vi "FreqC.Close Session.vi"(8 "error In":errorcluster, 11 "FreqC Session in":T1) -> (0 "error out":errorcluster)   [LabVIEW 2018]
uses:
  typedefs/FreqC.Session.ctl
  <instrlib>/Agilent 532XX Series/Agilent 532XX Series.lvlib
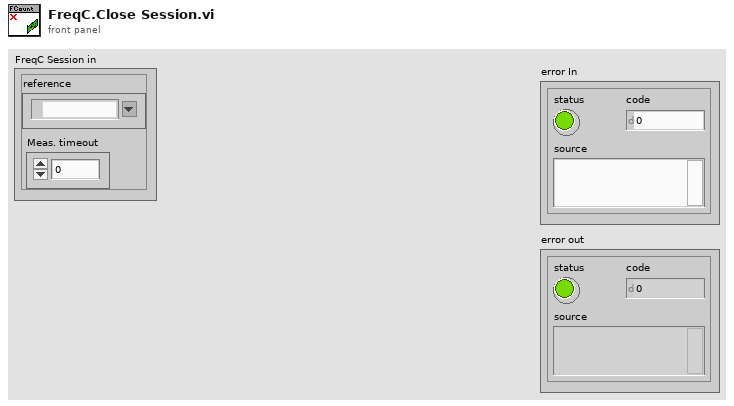
[diagram p1: front panel]
types:
  T1 = typedef "FreqC.Session.ctl" = cluster{"reference":refnum<visa-resource-name>, "Meas. timeout":dbl}
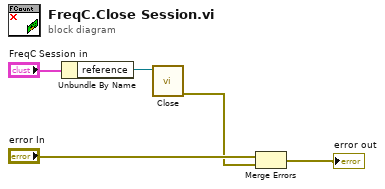
[diagram p0: block diagram]
diagram:
  n1 = Unbundle By Name("FreqC Session in") -> ("reference"=w4:refnum<visa-resource-name>)
  n2 = call <instrlib>:"Close.vi"("VISA resource name"=w4) -> ("error out"=w2:errorcluster)  [unwired: 10 in]
  n3 = Merge Errors("error In", w2) -> (→"error out":errorcluster)
